vi "Init File Ref.vi"(8 "error in":errorcluster) -> (0 "error out":errorcluster, 3 "Test Settings":refnum<file>)   [LabVIEW 2025, in "IT-M3900C.lvlib"]
uses:
  IT-M3900C.lvlib
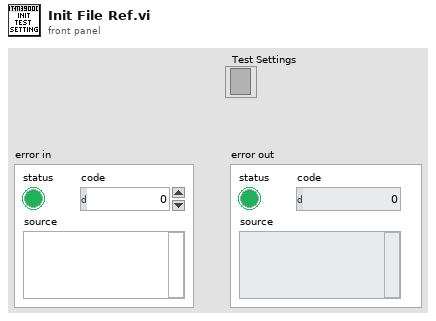
[diagram p1: front panel]
types:
  T1 = enum16{"open", "replace", "create", "open or create", "replace or create", "replace or create with confirmation"}
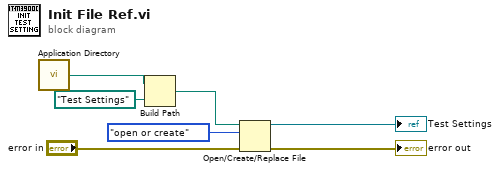
[diagram p0: block diagram]
diagram:
  n1 = call <vilib>:"Application Directory.vi"() -> ("Application Directory"=w4:path)
  n2 = Build Path(base path=w4, name or relative path=path "Test Settings") -> (appended path=w3:path)
  n3 = Open/Create/Replace File(file path (use dialog)=w3, error in="error in", operation (0:open)=T1."open or create") -> (refnum out=→"Test Settings":refnum<file>, error out=→"error out":errorcluster)  [unwired: 3 in, 1 out]
